vi "stop_B.vi"() -> ()   [LabVIEW 2013]
panel:
  in  "stop_B":bool
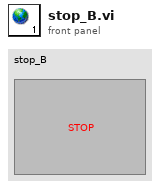
[diagram p1: front panel]
diagram:
